vi "Add SLSC Chassis.vi"(6 "SLSC Chassis Login":T1={"Username"="anonymous", "Password"=""}, 8 "error in (no error)":errorcluster, 9 "SLSC Chassis ID":T2 {"chassisType" items=["e12001_CHASSIS_TYPE"]; "ChassisIDType" items=["ChassisName", "HostnameIPAddress"]}, 10 "Target Name":string="Controller", 11 "SysDef in":refnum<k24>) -> (0 "error out":errorcluster, 2 "SLSC Chassis":u64, 3 "SysDef out":refnum<k24>)   [LabVIEW 2020, in "VeriStand SLSC Scripting.lvlib"]
uses:
  VeriStand SLSC Scripting.lvlib
  Controls/SLSC Chassis ID.ctl
  Controls/SLSC Chassis Login.ctl
  NationalInstruments.VeriStand.SystemDefinitionAPI
  NationalInstruments.VeriStand.SystemStorage
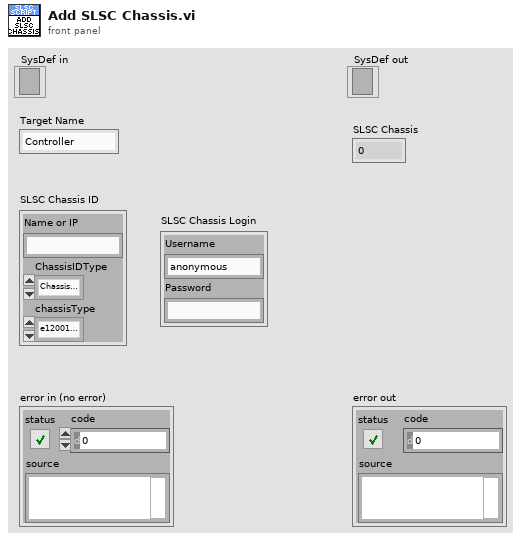
[diagram p1: front panel]
types:
  T1 = typedef "VeriStand SLSC Scripting.lvlib/SLSC Chassis Login.ctl" = cluster{"Username":string, "Password":string}
  T2 = typedef "VeriStand SLSC Scripting.lvlib/SLSC Chassis ID.ctl" = cluster{"Name or IP":string, "ChassisIDType":i32, "chassisType":i32}
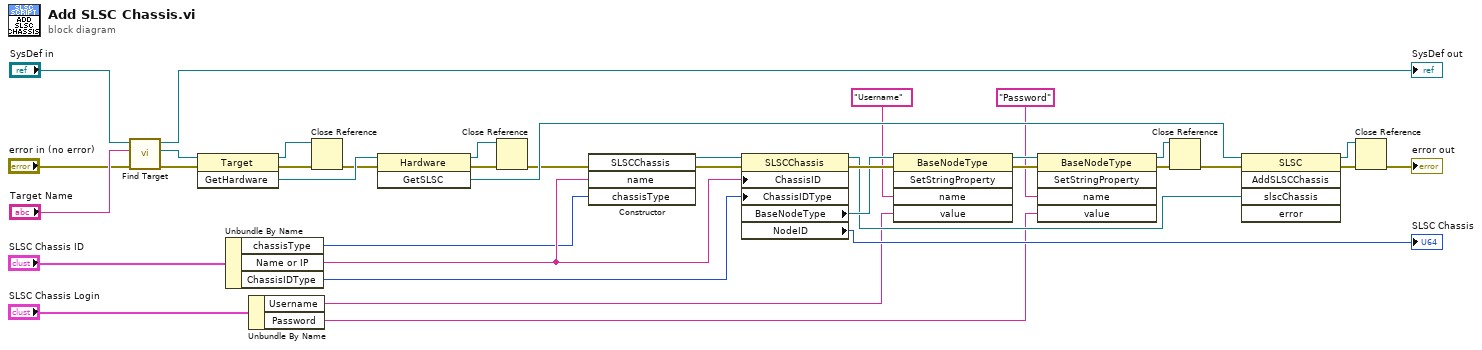
[diagram p0: block diagram]
diagram:
  n1 = call "Find Target.vi"("error in (no error)"="error in (no error)", "Name"="Target Name", "SysDef in"="SysDef in") -> ("error out"=w4:errorcluster, "Target"=w6:refnum<k24>, "SysDef out"=→"SysDef out":refnum<k24>)  [unwired: 6 in]
  n2 = invoke class="Target" method="GetHardware"(reference=w6, error in=w4) -> (reference out=w1:refnum<k24>, error out=w36:errorcluster, "GetHardware"=w37:refnum<k24>)  [unwired: 1 in]
  n3 = Unbundle By Name("SLSC Chassis ID") -> ("chassisType"=w3:i32, "Name or IP"=w13:string, "ChassisIDType"=w12:i32)
  n4 = Unbundle By Name("SLSC Chassis Login") -> ("Username"=w11:string, "Password"=w10:string)
  n5 = Close Reference(reference=w1, error in (no error)=w36) -> (error out=w2:errorcluster)
  n6 = invoke class="Hardware" method="GetSLSC"(reference=w37, error in=w2) -> (reference out=w32:refnum<k24>, error out=w34:errorcluster, "GetSLSC"=w35:refnum<k24>)  [unwired: 1 in]
  n7 = Close Reference(reference=w32, error in (no error)=w34) -> (error out=w33:errorcluster)
  n8 = constructor class="SLSCChassis"(error in=w33, "name"=w13, "chassisType"=w3) -> (reference out=w30:refnum<k24>, error out=w31:errorcluster)  [unwired: 2 in, 3 out]
  n9 = property class="SLSCChassis"(reference=w30, error in=w31, "ChassisID"=w13, "ChassisIDType"=w12) -> (reference out=w17:refnum<k24>, error out=w29:errorcluster, "BaseNodeType"=w28:refnum<k24>, "NodeID"=→"SLSC Chassis":u64)
  n10 = invoke class="BaseNodeType" method="SetStringProperty"(reference=w28, error in=w29, "name"="Username", "value"=w11) -> (reference out=w26:refnum<k24>, error out=w27:errorcluster)  [unwired: 1 in, 3 out]
  n11 = invoke class="BaseNodeType" method="SetStringProperty"(reference=w26, error in=w27, "name"="Password", "value"=w10) -> (reference out=w21:refnum<k24>, error out=w23:errorcluster)  [unwired: 1 in, 3 out]
  n12 = Close Reference(reference=w21, error in (no error)=w23) -> (error out=w22:errorcluster)
  n13 = invoke class="SLSC" method="AddSLSCChassis"(reference=w35, error in=w22, "slscChassis"=w17) -> (reference out=w18:refnum<k24>, error out=w20:errorcluster)  [unwired: 2 in, 3 out]
  n14 = Close Reference(reference=w18, error in (no error)=w20) -> (error out=→"error out":errorcluster)
